vi "Read Application Style Reference.vi"(11 "IViewable in":refnum<class "IViewable.lvclass">) -> (2 "Application Style Reference":T1)   [LabVIEW 2017, in "IViewable.lvlib" / "IViewable.lvclass"]
uses:
  IViewable.lvclass
  ApplicationStyleReference/Application Style Reference.ctl
  ApplicationStyleReference/ApplicationStyleReference.lvclass
  IViewable.lvclass/IViewable.ctl
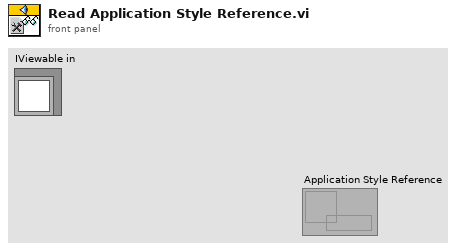
[diagram p1: front panel]
types:
  T1 = typedef "IViewable.lvlib/ApplicationStyleReference.lvclass/Application Style Reference.ctl" = refnum<data-value>
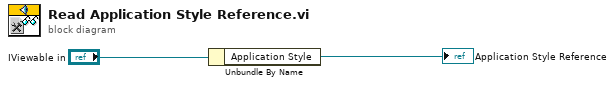
[diagram p0: block diagram]
diagram:
  n1 = Unbundle By Name("IViewable in") -> ("Application Style"=→"Application Style Reference":T1)
